vi "Output Level to Volts.vi"(10 "Output level in":dbl, 11 "Output level units":string) -> (3 "Output level out":dbl)   [LabVIEW 2021]
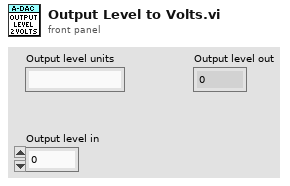
[diagram p1: front panel]
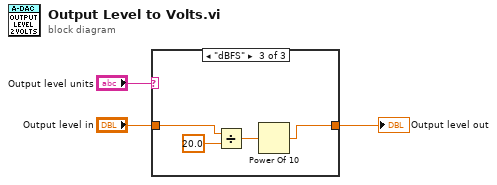
[diagram p0: block diagram]
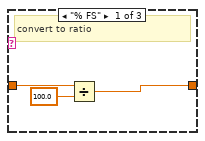
[diagram p2: hidden frame]
diagram:
  n1 = case shown="\"dBFS\"" "Output level units" {
    tunnel: "Output level in" -> [w6 w7 w9]
    tunnel: [w4 w7 w8] -> w2
    frame "% FS" {
      # "convert to ratio"
      n2 = Divide(x=w6, y=100.0) -> (x/y=w4:dbl)
    }
    frame "V", Default {
      # "no conversion"
    }
    frame "dBFS" {
      n3 = Divide(x=w9, y=20.0) -> (x/y=w11:dbl)
      n4 = Power Of 10(x=w11) -> (10^x=w8:dbl)
    }
  }
  "Output level out" <- w2
